vi "gRPC Client Test.vi"() -> ()   [LabVIEW 2021, in "NI Switch_client.lvlib"]
uses:
  NI Switch_client.lvlib
  RPC Messages/nidevice_grpc_SessionInitializationBehavior.ctl
  RPC Messages/niswitch_grpc_InitWithTopologyRequest.ctl
  <vilib>/Plug-In SDKs/Clients/Discovery V1/NI Discovery V1 Client.lvlib
  <vilib>/gRPC/Generated APIs/ni/measurementlink/discovery/v1/RPC Messages/ni_measurementlink_discovery_v1_ResolveServiceRequest.ctl
  <vilib>/gRPC/Generated APIs/ni/measurementlink/discovery/v1/ni.measurementlink.discovery.v1.api.lvlib
  RPC Messages/nidevice_grpc_Session.ctl
  RPC Messages/niswitch_grpc_CloseRequest.ctl
  RPC Messages/niswitch_grpc_InitWithTopologyResponse.ctl
  RPC Messages/niswitch_grpc_CloseResponse.ctl
panel:
  out "Client 2 Init Response":T1
  out "Close Response":T3
  out "Client 1 Init Response":T1
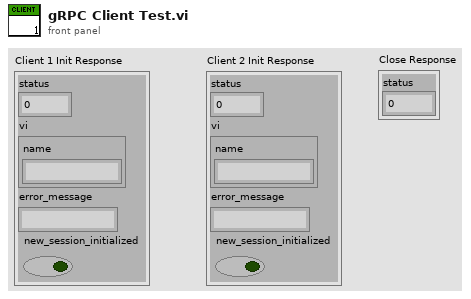
[diagram p1: front panel]
types:
  T1 = typedef "NI Switch_client.lvlib/niswitch_grpc_InitWithTopologyResponse.ctl" = cluster{"status":i32, "vi":T2, "error_message":string, "new_session_initialized":bool}
  T2 = typedef "NI Switch_client.lvlib/nidevice_grpc_Session.ctl" = cluster{"name":string}
  T3 = typedef "NI Switch_client.lvlib/niswitch_grpc_CloseResponse.ctl" = cluster{"status":i32}
  T4 = typedef "NI Switch_client.lvlib/niswitch_grpc_CloseRequest.ctl" = cluster{"vi":T2}
  T5 = typedef "NI Switch_client.lvlib/nidevice_grpc_SessionInitializationBehavior.ctl" = enum32{"SESSION_INITIALIZATION_BEHAVIOR_UNSPECIFIED", "SESSION_INITIALIZATION_BEHAVIOR_INITIALIZE_NEW", "SESSION_INITIALIZATION_BEHAVIOR_ATTACH_TO_EXISTING"}
  T6 = typedef "ni.measurementlink.discovery.v1.api.lvlib/ni_measurementlink_discovery_v1_ResolveServiceRequest.ctl" = cluster{"provided_interface":string, "service_class":string, "deployment_target":string, "version":string}
  T7 = typedef "NI Switch_client.lvlib/niswitch_grpc_InitWithTopologyRequest.ctl" = cluster{"session_name":string, "resource_name":string, "topology":string, "simulate":bool, "reset_device":bool, "initialization_behavior":T5}
  T8 = typedef "ni.measurementlink.discovery.v1.api.lvlib/ni_measurementlink_discovery_v1_ServiceLocation.ctl" = cluster{"location":string, "insecure_port":string, "ssl_authenticated_port":string}
  T9 = typedef "grpc-lvsupport-release.lvlib/grpcId.ctl" = u64
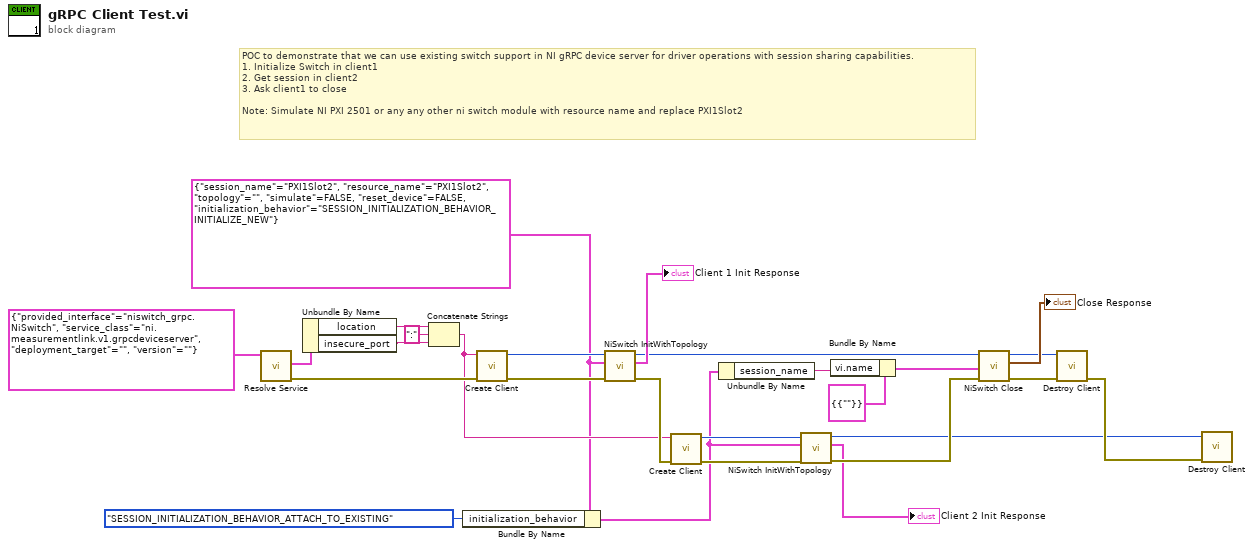
[diagram p0: block diagram]
diagram:
  w6 = T7 {"session_name"="PXI1Slot2", "resource_name"="PXI1Slot2", "topology"="", "simulate"=FALSE, "reset_device"=FALSE, "initialization_behavior"=enum."SESSION_INITIALIZATION_BEHAVIOR_INITIALIZE_NEW"} ("Request Data")
  # "POC to demonstrate that we can use existing switch support in NI gRPC device server for driver operations with session sharing capabilities.\n1. Initialize Switch in client1\n2. Get session in client2\n3. Ask client1 to close\n\nNote: Simulate NI PXI 2501 or any any other ni switch module with resource name and replace PXI1Slot2"
  n1 = call <vilib>:"Resolve Service.vi"("request data"=T6 {"provided_interface"="niswitch_grpc.NiSwitch", "service_class"="ni.measurementlink.v1.grpcdeviceserver", "deployment_target"="", "version"=""}) -> ("error out"=w11:errorcluster, "response data"=w12:T8)  [unwired: 9 in]
  n2 = Unbundle By Name(w12) -> ("location"=w10:string, "insecure_port"=w9:string)
  n3 = Concatenate Strings(w10, ":" ("string"), w9) -> (w7:string)
  n4 = Bundle By Name(cluster=w6, "initialization_behavior"=nidevice_grpc_SessionInitializationBehavior."SESSION_INITIALIZATION_BEHAVIOR_ATTACH_TO_EXISTING") -> (w4:T7)
  n5 = call "Create Client.vi"("error in"=w11, "address"=w7) -> ("error out"=w26:errorcluster, "gRPC ID Out"=w27:T9)  [unwired: 8 in]
  n6 = call "NiSwitch InitWithTopology.vi"("error in"=w26, "Request Data"=w6, "gRPC ID"=w27) -> ("error out"=w22:errorcluster, "Response Data"=→"Client 1 Init Response":T1, "gRPC ID out"=w14:T9)  [unwired: 6 in]
  n7 = call "Create Client.vi"("error in"=w22, "address"=w7) -> ("error out"=w24:errorcluster, "gRPC ID Out"=w23:T9)  [unwired: 8 in]
  n8 = Unbundle By Name(w4) -> ("session_name"=w1:string)
  n9 = call "NiSwitch InitWithTopology.vi"("error in"=w24, "Request Data"=w4, "gRPC ID"=w23) -> ("error out"=w20:errorcluster, "Response Data"=→"Client 2 Init Response":T1, "gRPC ID out"=w16:T9)  [unwired: 6 in]
  n10 = Bundle By Name(cluster=T4 {"vi"={"name"=""}} ("Request Data"), "vi.name"=w1) -> (w2:T4)
  n11 = call "NiSwitch Close.vi"("error in"=w20, "Request Data"=w2, "gRPC ID"=w14) -> ("error out"=w19:errorcluster, "Response Data"=→"Close Response":T3, "gRPC ID out"=w15:T9)  [unwired: 6 in]
  n12 = call "Destroy Client.vi"("error in"=w19, "gRPC ID"=w15) -> ("error out"=w21:errorcluster)  [unwired: 9 in]
  n13 = call "Destroy Client.vi"("error in"=w21, "gRPC ID"=w16) -> ()  [unwired: 9 in, 1 out]
